vi "Coaxial_PID_Encoder_6.vi"() -> ()   [LabVIEW 2022 SP3]
uses:
  <vilib>/DAQmx/read.llb/DAQmx Read (Counter DBL 1Chan 1Samp).vi
  <vilib>/DAQmx/write.llb/DAQmx Write (Counter 1D Frequency NChan 1Samp).vi
  <vilib>/DAQmx/create/channels.llb/DAQmx Create Channel (CO-Pulse Generation-Frequency).vi
  <vilib>/DAQmx/configure/timing.llb/DAQmx Timing (Implicit).vi
  <vilib>/DAQmx/create/channels.llb/DAQmx Create Channel (CI-Count Edges).vi
  <vilib>/DAQmx/miscellaneous.llb/DAQmx Fill In Error Info.vi
  <vilib>/addons/control/pid/NI_PID_autopid.lvlib
  <vilib>/ptbypt/NI_PtbyPt.lvlib
  <resource>/objmgr/daqmx.rc
panel:
  out "number of samples written per channel":u32
  out "Array":cluster{dbl, "element":dbl}[](array[cluster])
  out "PWM upper":dbl
  in  "PID gains 2":T1={"proportional gain (Kc)"=0.002855, "integral time (Ti, min)"=0.003704, "derivative time (Td, min)"=0.000926} {"derivative time (Td, min)" format="%.6f"; "integral time (Ti, min)" format="%.6f"; "proportional gain (Kc)" format="%.6f"}
  in  "output range 2":cluster{"output high":dbl, "output low":dbl}={"output high"=2000.0, "output low"=1000.0} {"output low" format="%.2f"; "output high" format="%.2f"}
  in  "counter 3":tag="Dev2/ctr0"
  in  "edge":i32(ring)=10280 items=["Rising"=10280, "Falling"=10171]
  in  "samples per channel":i32=1000
  in  "duty cycle":dbl=0.5 format="%.6f"
  in  "frequency":dbl=500.0 format="%.6f"
  in  "counter 2":tag="Dev2/ctr2"
  in  "counter":tag="Dev2/ctr3"
  out "RPM":dbl
  in  "stop":bool
  out "ti":dbl=1.3078203201293945
  out "ti-1":dbl=1.2584419250488281
  out "dt 2":dbl=0.049378395080566406
  in  "milliseconds to wait":u32=50
  in  "PID gains":T1={"proportional gain (Kc)"=0.002855, "integral time (Ti, min)"=0.003704, "derivative time (Td, min)"=0.000926} {"derivative time (Td, min)" format="%.6f"; "integral time (Ti, min)" format="%.6f"; "proportional gain (Kc)" format="%.6f"}
  in  "sample length for avg RPM":i32=5
  out "RPM Mov_Avg":dbl
  out "Mov_Avg RPM":dbl(graph)
  out "PWM 2":dbl=0.5
  out "dt":dbl(graph)=0.049378395080566406
  out "Achieved RPM 2":dbl(graph)
  in  "Position control on/off":bool
  out "position control output setpoint":dbl
  in  "Time Target (s)":dbl=10.0
  in  "Angle SetPoint (deg)":dbl
  out "Elapsed Reset time (s)":dbl caption="Elapsed Time (s)"
  in  "?":dbl
  in  "pos change speed":dbl=3000.0
  in  "setpoint 2":dbl format="%.2f"
  out "RPM 2":dbl
  out "Achieved RPM":dbl(graph)
  out "RPM Mov_Avg 2":dbl
  out "Mov_Avg RPM  2":dbl(graph)
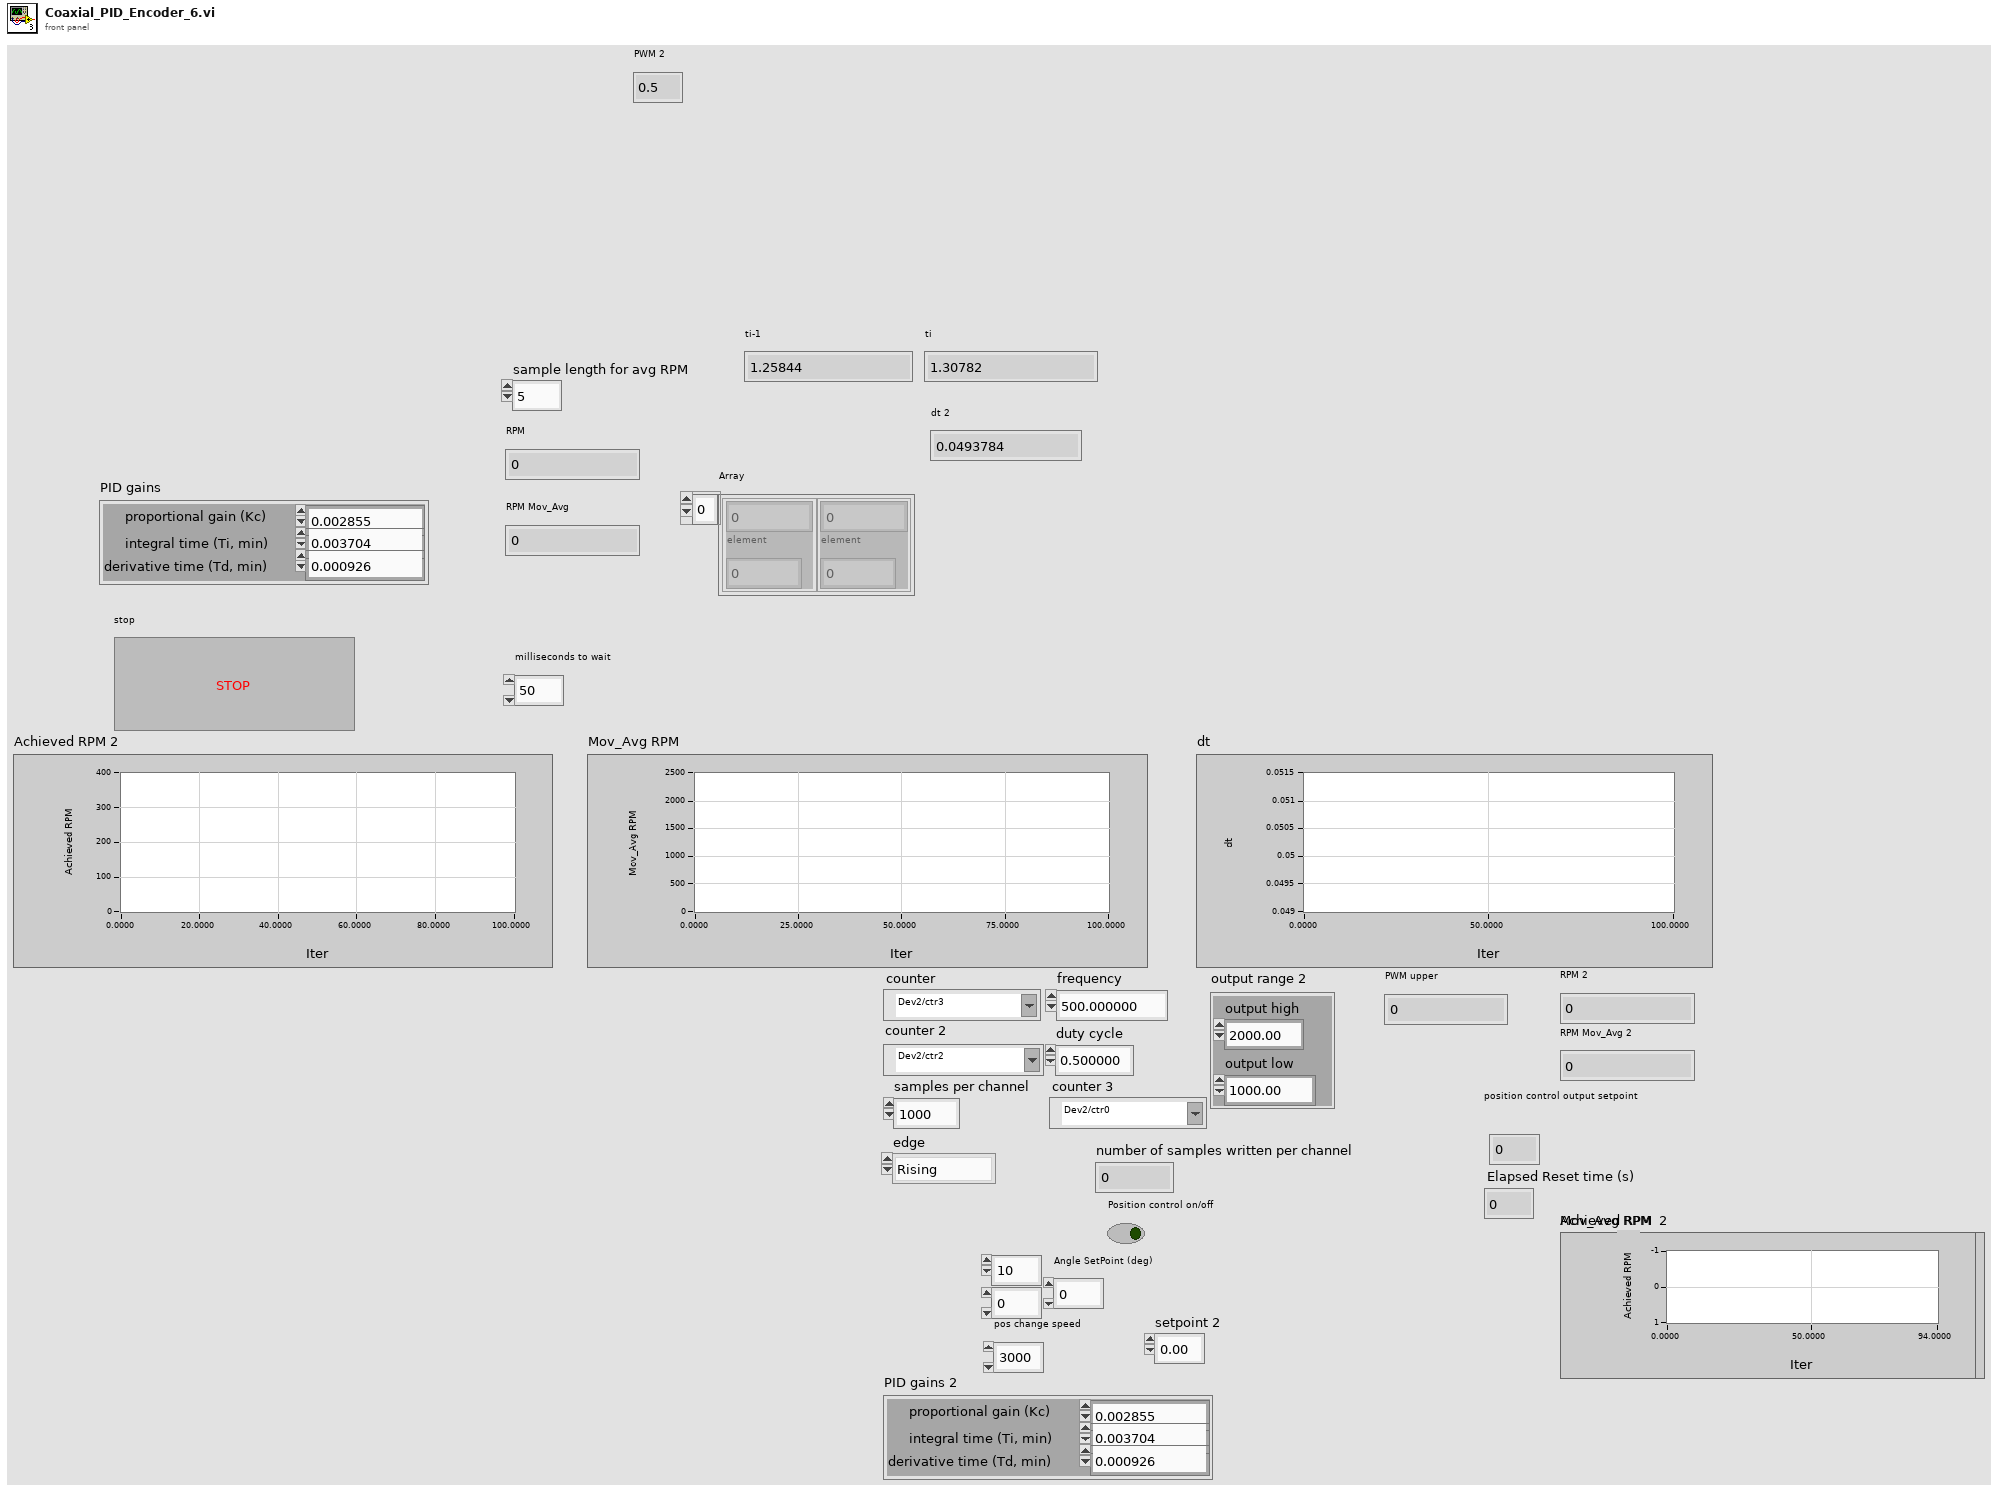
[diagram p1: front panel]
types:
  T1 = cluster{"proportional gain (Kc)":dbl, "integral time (Ti, min)":dbl, "derivative time (Td, min)":dbl}
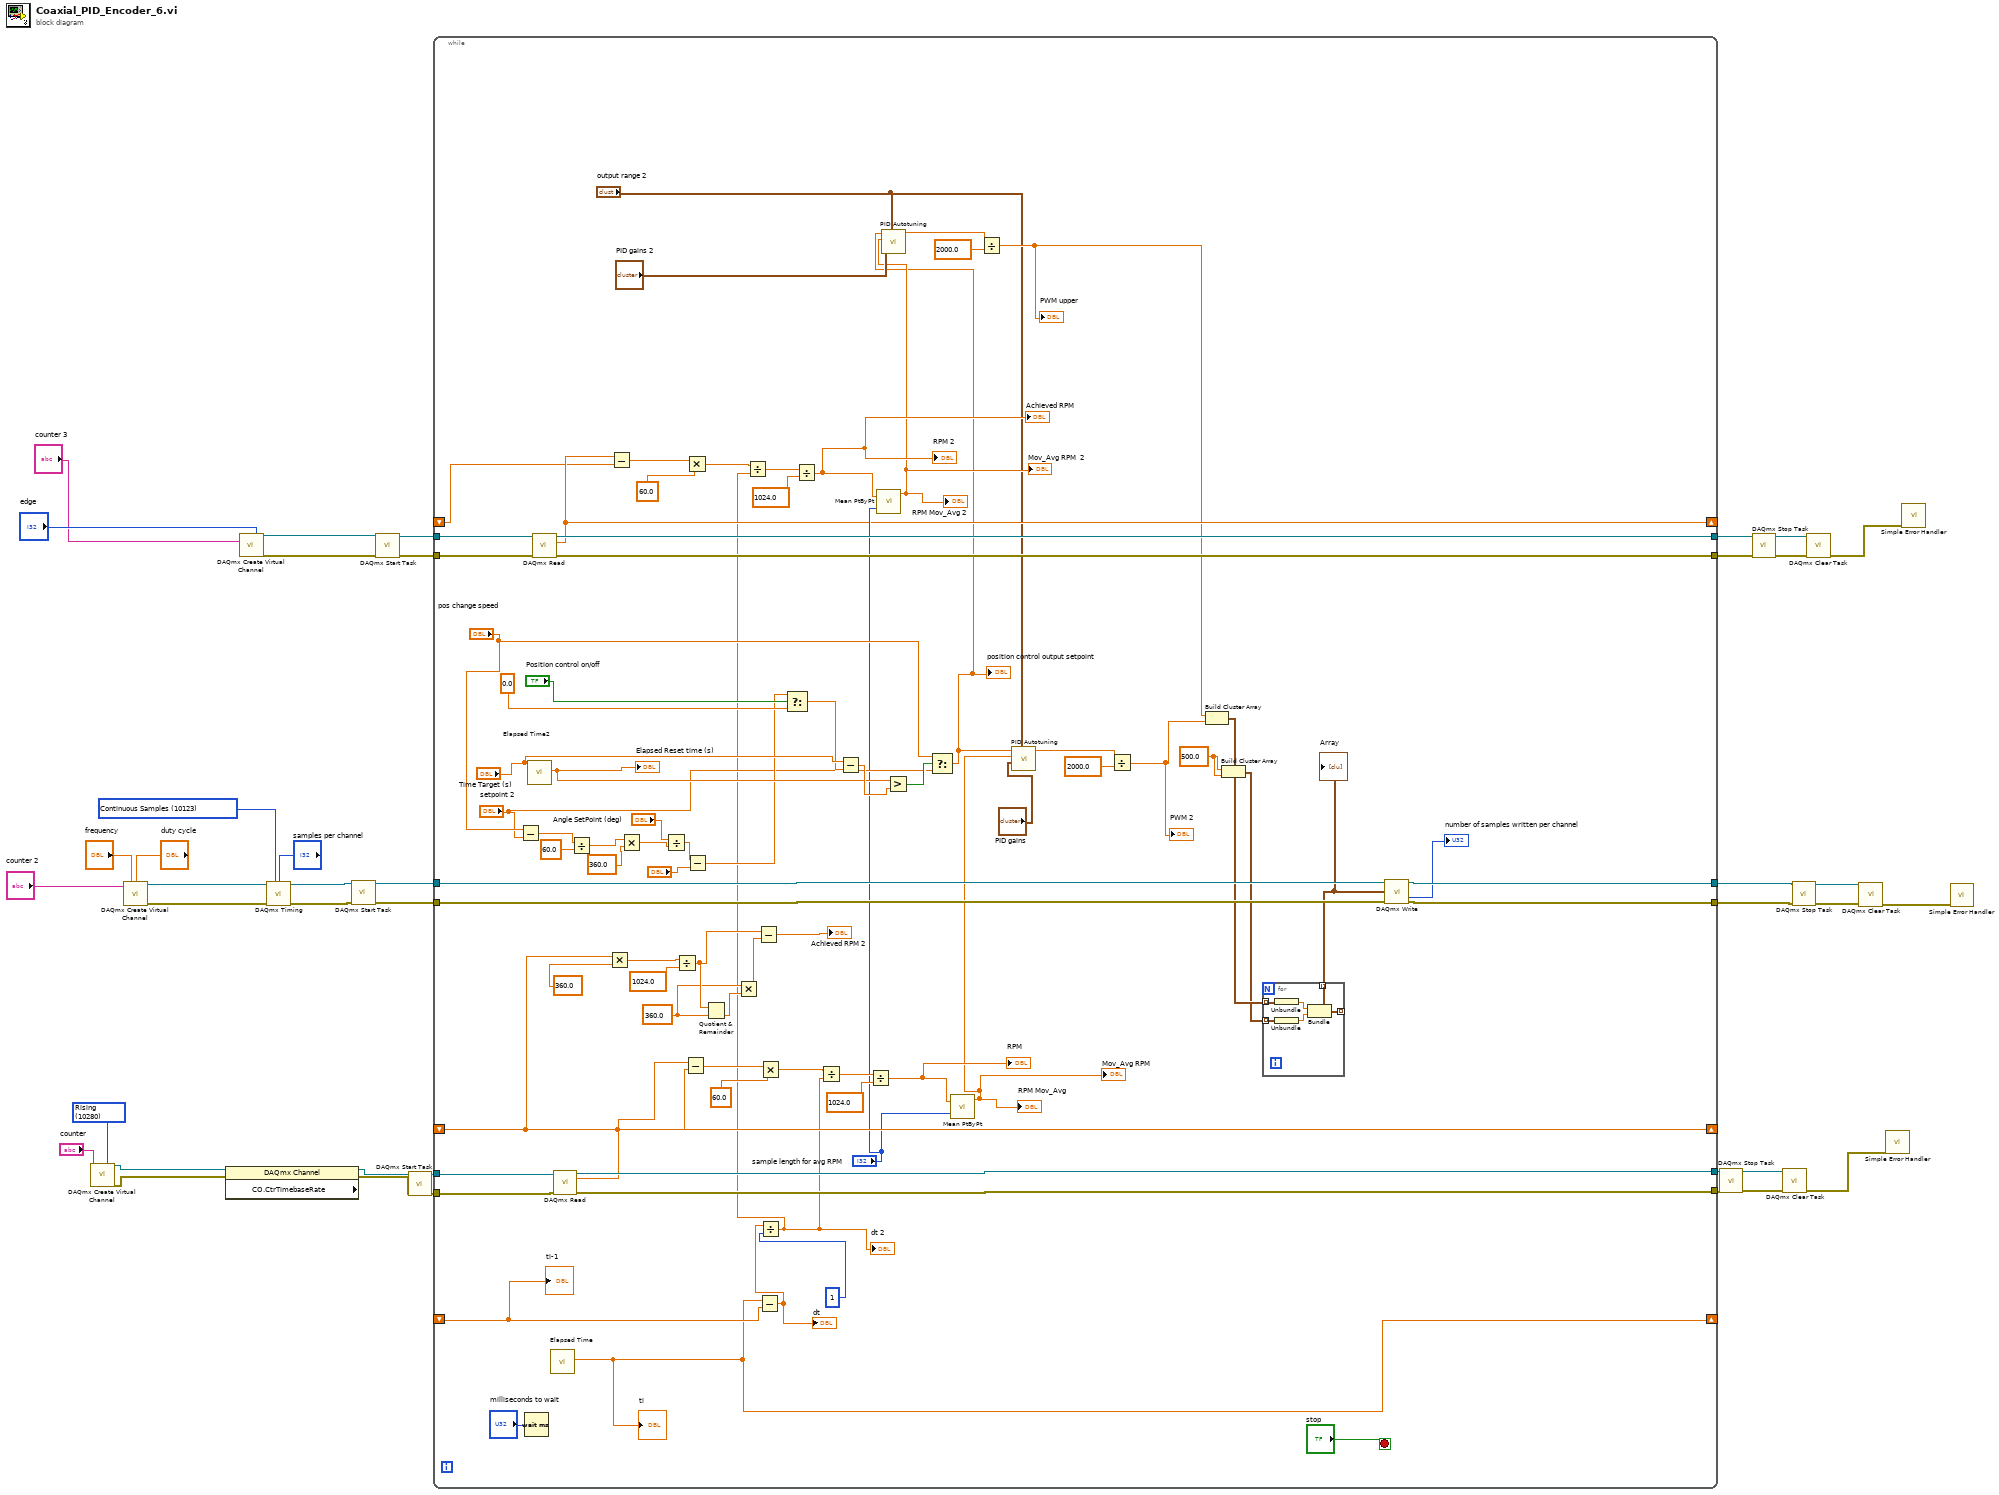
[diagram p0: block diagram]
diagram:
  w16 = 10280 items=["Rising"=10280, "Falling"=10171] ("edge")
  w24 = 10123 items=["Finite Samples"=10178, "Continuous Samples"=10123, "Hardware Timed Single Point"=12522] ("sample mode")
  n1 = call-poly <vilib>:"DAQmx Create Virtual Channel.vi"("edge"=w16, "counter"="counter") -> ("task out"=w15:refnum<k21>, "error out"=w14:errorcluster)  [unwired: 12 in]
  n2 = call-poly <vilib>:"DAQmx Create Virtual Channel.vi"("frequency"="frequency", "duty cycle"="duty cycle", "counter"="counter 2") -> ("task out"=w32:refnum<k21>, "error out"=w30:errorcluster)  [unwired: 11 in]
  n3 = property class="DAQmx Channel" props=["CO.CtrTimebaseRate"](reference=w15, error in=w14) -> (reference out=w13:refnum<k21>, error out=w12:errorcluster)  [unwired: 1 out]
  n4 = call-poly <vilib>:"DAQmx Create Virtual Channel.vi"("edge"="edge", "counter"="counter 3") -> ("task out"=w9:refnum<k21>, "error out"=w8:errorcluster)  [unwired: 12 in]
  n5 = call-poly <vilib>:"DAQmx Timing.vi"("task/channels in"=w32, "sample mode"=w24, "samples per channel"="samples per channel", "error in"=w30) -> ("task out"=w31:refnum<k21>, "error out"=w29:errorcluster)  [unwired: 10 in]
  n6 = call <vilib>:"DAQmx Start Task.vi"("task/channels in"=w31, "error in"=w29) -> ("task out"=w20:refnum<k21>, "error out"=w19:errorcluster)  [unwired: 12 in]
  n7 = call <vilib>:"DAQmx Start Task.vi"("task/channels in"=w9, "error in"=w8) -> ("task out"=w7:refnum<k21>, "error out"=w6:errorcluster)  [unwired: 12 in]
  n8 = call <vilib>:"DAQmx Start Task.vi"("task/channels in"=w13, "error in"=w12) -> ("task out"=w40:refnum<k21>, "error out"=w39:errorcluster)  [unwired: 12 in]
  n9 = while {
    tunnel: w40 -> [w119]
    tunnel: w39 -> [w118]
    tunnel: [w117] -> w38
    tunnel: [w116] -> w37
    shift-right: [w109] -> _
    shift-left: _ -> [w88]
    shift-right: [w106] -> _
    shift-left: _ -> [w108]
    tunnel: w20 -> [w105]
    tunnel: w19 -> [w104]
    tunnel: [w103] -> w18
    tunnel: [w102] -> w17
    tunnel: w7 -> [w68]
    tunnel: w6 -> [w67]
    tunnel: [w66] -> w2
    tunnel: [w65] -> w1
    shift-right: [w57] -> _
    shift-left: _ -> [w56]
    stop <- "stop" stop-if-true
    w48 = 500.0 ("element")
    w89 = 360.0 ("y")
    n10 = Subtract(x="pos change speed", y="setpoint 2") -> (x-y=w74:dbl)
    n11 = Wait (ms)(milliseconds to wait="milliseconds to wait") -> ()  [unwired: 1 out]
    n12 = call "Elapsed Time2"("Time Target (s)"="Time Target (s)") -> ("Elapsed Time (s)"=w80:dbl)  [unwired: 11 in, 7 out]
    "Elapsed Reset time (s)" <- w80
    n13 = call-poly <vilib>:"DAQmx Read.vi"("task/channels in"=w68, "error in"=w67) -> ("task out"=w66:refnum<k21>, "data"=w57:dbl, "error out"=w65:errorcluster)  [unwired: 11 in]
    n14 = call "Elapsed Time"() -> ("Elapsed Time (s)"=w106:dbl)  [unwired: 12 in, 7 out]
    "ti" <- w106
    n15 = call-poly <vilib>:"DAQmx Read.vi"("task/channels in"=w119, "error in"=w118) -> ("task out"=w117:refnum<k21>, "data"=w109:dbl, "error out"=w116:errorcluster)  [unwired: 11 in]
    n16 = Divide(x=w74, y=60.0) -> (x/y=w78:dbl)
    n17 = Multiply(x=w88, y=360.0) -> (x*y=w94:dbl)
    n18 = Subtract(x=w57, y=w56) -> (x-y=w60:dbl)
    n19 = Multiply(x=w78, y=360.0) -> (x*y=w76:dbl)
    n20 = Divide(x="Angle SetPoint (deg)", y=w76) -> (x/y=w73:dbl)
    n21 = Divide(x=w94, y=1024.0) -> (x/y=w91:dbl)
    n22 = Subtract(x=w109, y=w88) -> (x-y=w98:dbl)
    n23 = Multiply(x=w60, y=60.0) -> (x*y=w63:dbl)
    n24 = Subtract(x=w73, y="?") -> (x-y=w72:dbl)
    n25 = Quotient & Remainder(x=w91, y=w89) -> (floor(x/y)=w90:dbl)  [unwired: 1 out]
    n26 = Multiply(x=w89, y=w90) -> (x*y=w92:dbl)
    n27 = Subtract(x=w91, y=w92) -> (x-y=→"Achieved RPM 2":dbl)
    n28 = Subtract(x=w106, y=w108) -> (x-y=w97:dbl)
    "dt" <- w97
    n29 = Multiply(x=w98, y=60.0) -> (x*y=w114:dbl)
    n30 = Divide(x=w97, y=u32 1) -> (x/y=w55:dbl)
    "dt 2" <- w55
    n31 = Divide(x=w63, y=w55) -> (x/y=w62:dbl)
    n32 = Select(t=w72, s="Position control on/off", f=0.0) -> (s? t:f=w81:dbl)
    n33 = Divide(x=w62, y=1024.0) -> (x/y=w59:dbl)
    "RPM 2" <- w59
    "Achieved RPM" <- w59
    n34 = Divide(x=w114, y=w55) -> (x/y=w113:dbl)
    n35 = Subtract(x="Time Target (s)", y=w81) -> (x-y=w83:dbl)
    n36 = Divide(x=w113, y=1024.0) -> (x/y=w99:dbl)
    "RPM" <- w99
    n37 = call <vilib>:"Mean PtByPt.vi"("x"=w59, "sample length"="sample length for avg RPM") -> ("mean"=w51:dbl)  [unwired: 2 in, 1 out]
    "RPM Mov_Avg 2" <- w51
    "Mov_Avg RPM  2" <- w51
    n38 = Greater?(x=w80, y=w83) -> (0:w84:bool)
    n39 = Select(t="pos change speed", s=w84, f="setpoint 2") -> (s? t:f=w41:dbl)
    "position control output setpoint" <- w41
    n40 = call <vilib>:"PID Autotuning.vi"("output range"="output range 2", "PID gains"="PID gains 2", "process variable"=w51, "setpoint"=w41) -> ("output"=w53:dbl)  [unwired: 4 in, 3 out]
    n41 = call <vilib>:"Mean PtByPt.vi"("x"=w99, "sample length"="sample length for avg RPM") -> ("mean"=w96:dbl)  [unwired: 2 in, 1 out]
    "RPM Mov_Avg" <- w96
    "Mov_Avg RPM" <- w96
    n42 = Divide(x=w53, y=2000.0) -> (x/y=w49:dbl)
    "PWM upper" <- w49
    n43 = call <vilib>:"PID Autotuning.vi"("output range"="output range 2", "PID gains"="PID gains", "process variable"=w96, "setpoint"=w41) -> ("output"=w50:dbl)  [unwired: 4 in, 3 out]
    n44 = Divide(x=w50, y=2000.0) -> (x/y=w45:dbl)
    "PWM 2" <- w45
    n45 = Build Cluster Array(w49, w45) -> (w47:cluster{dbl}[])
    n46 = Build Cluster Array(w48, w48) -> (w46:cluster{"element":dbl}[])
    n47 = for {
      tunnel: w47 -> [w124] mode=indexing
      tunnel: w46 -> [w123] mode=indexing
      tunnel: [w120] -> _ mode=indexing
      tunnel: [w120] -> w43 mode=indexing
      n48 = Unbundle(w124) -> (w122:dbl)
      n49 = Unbundle(w123) -> ("element"=w121:dbl)
      n50 = Bundle(w122, "element"=w121) -> (w120:cluster{dbl, "element":dbl})  [unwired: 1 out]
    }
    "Array" <- w43
    n51 = call-poly <vilib>:"DAQmx Write.vi"("task/channels in"=w105, "data"=w43, "error in"=w104) -> ("task out"=w103:refnum<k21>, "number of samples written per channel"=→"number of samples written per channel":u32, "error out"=w102:errorcluster)  [unwired: 10 in]
    "ti-1" <- w108
  }
  n52 = call <vilib>:"DAQmx Stop Task.vi"("task/channels in"=w38, "error in"=w37) -> ("task out"=w36:refnum<k21>, "error out"=w35:errorcluster)  [unwired: 12 in]
  n53 = call <vilib>:"DAQmx Stop Task.vi"("task/channels in"=w2, "error in"=w1) -> ("task out"=w5:refnum<k21>, "error out"=w4:errorcluster)  [unwired: 12 in]
  n54 = call <vilib>:"DAQmx Clear Task.vi"("task in"=w36, "error in"=w35) -> ("error out"=w34:errorcluster)  [unwired: 13 in]
  n55 = call <vilib>:"DAQmx Stop Task.vi"("task/channels in"=w18, "error in"=w17) -> ("task out"=w23:refnum<k21>, "error out"=w22:errorcluster)  [unwired: 12 in]
  n56 = call <vilib>:"DAQmx Clear Task.vi"("task in"=w5, "error in"=w4) -> ("error out"=w3:errorcluster)  [unwired: 13 in]
  n57 = call <vilib>:"DAQmx Clear Task.vi"("task in"=w23, "error in"=w22) -> ("error out"=w21:errorcluster)  [unwired: 13 in]
  n58 = call <vilib>:"Simple Error Handler.vi"("error in (no error)"=w34) -> ()  [unwired: 4 in, 5 out]
  n59 = call <vilib>:"Simple Error Handler.vi"("error in (no error)"=w3) -> ()  [unwired: 4 in, 5 out]
  n60 = call <vilib>:"Simple Error Handler.vi"("error in (no error)"=w21) -> ()  [unwired: 4 in, 5 out]
